vi "EnFlo_Data_Sync_Manual.vi"() -> ()   [LabVIEW 2013]
uses:
  Anemometry Sub Vis/Controls/EnFlo_Data_Folder_Setup.ctl
  ADAM Client/Sub VIs/Harvest_Global.vi
  Anemometry Sub Vis/Globals/Preference_global.vi
  Anemometry Sub Vis/Globals/Constants_global.vi
panel:
  in  "stop":bool
  out "Currrently Pulled":i32
  out "No Files to Push":i32
  out "No Files to Pull":i32
  out "Currrently Pushed":i32
  out "File being transfered":path
  out "Currently":string
  out "Files to Pull From Server":path[](array[path])
  out "Files to Push to Server":path[](array[path])
  in  "Browse Remote Disk":bool
  out "error out":errorcluster
  out "Folder contents changed?":bool
  in  "Folder to Sync (Must be within Local EnFlo Data)":path=path "C:/EnFlo_Data_Temp/EnFlo_Software_SVN"
  in  "Get all Server Files":bool
  in  "Check Updates on Server?":bool
  in  "Archive Files?":bool
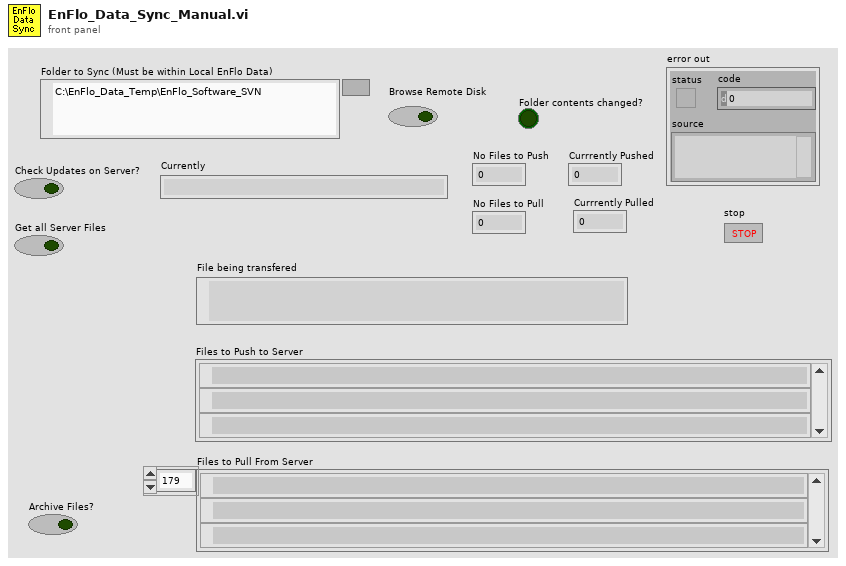
[diagram p1: front panel]
types:
  T1 = typedef "EnFlo_Data_Folder_Setup.ctl" = string
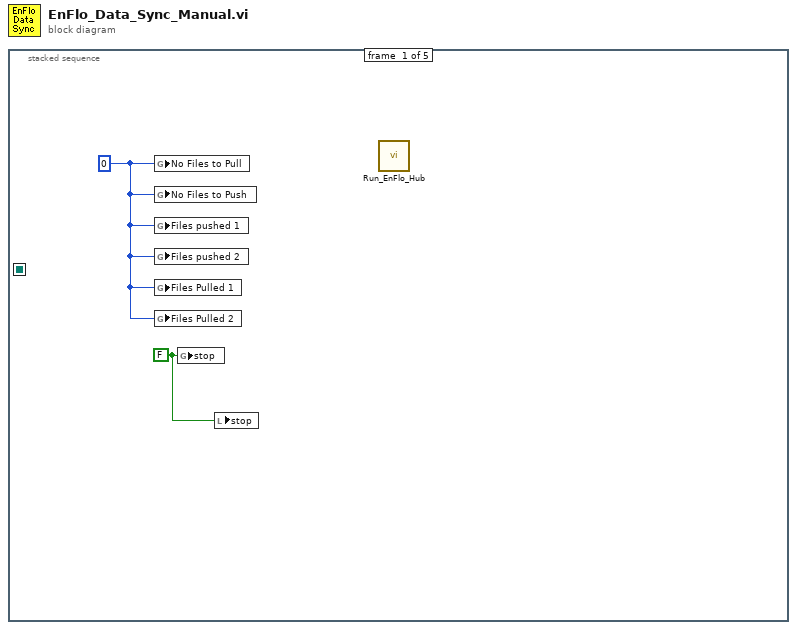
[diagram p0: block diagram]
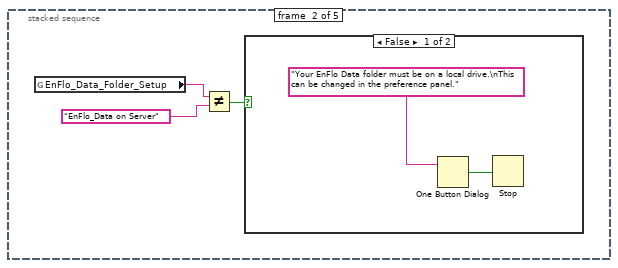
[diagram p2: hidden frame]
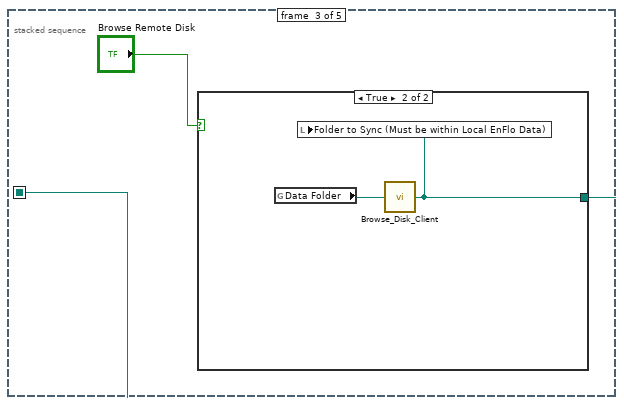
[diagram p4: hidden frame]
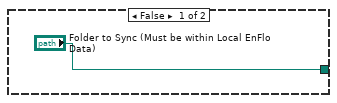
[diagram p5: hidden frame]
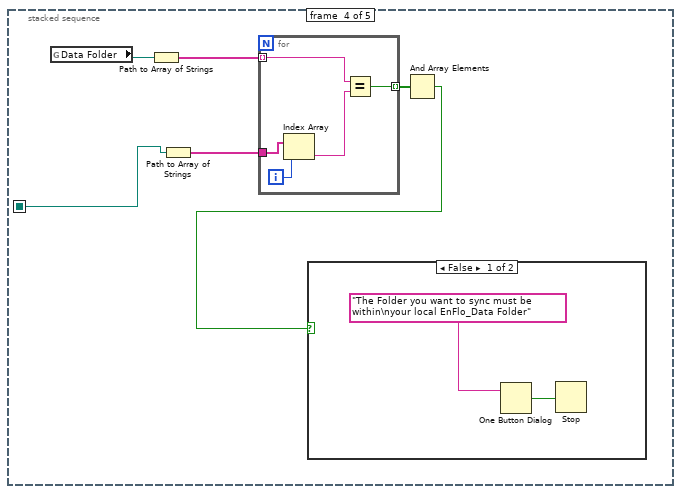
[diagram p6: hidden frame]
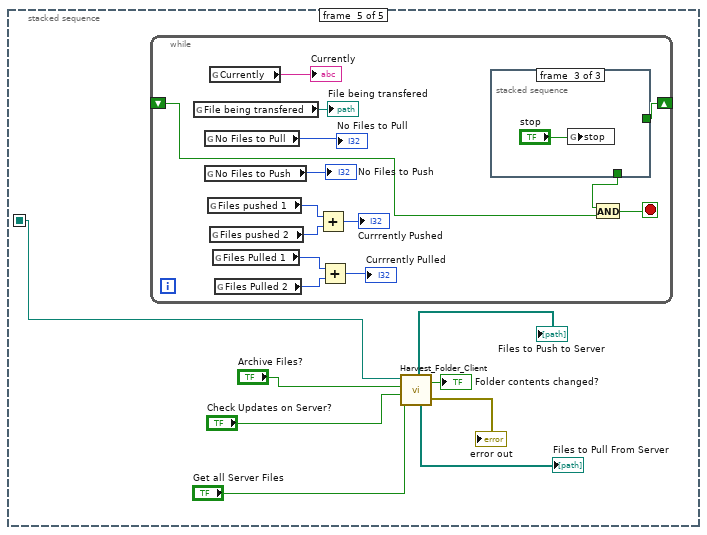
[diagram p8: hidden frame]
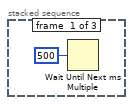
[diagram p9: hidden frame]
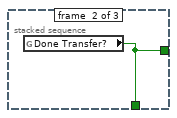
[diagram p10: hidden frame]
diagram:
  n1 = stacked-sequence {
    seq-local: [_ _ w8 _ _] -> [_ _ _ w13 w28]
    frame #0 {
      w1 = FALSE ("stop")
      w2 = 0 ("No Files to Pull")
      n2 = global write "Harvest_Global.vi" "No Files to Pull"(w2) -> ()
      n3 = global write "Harvest_Global.vi" "No Files to Push"(w2) -> ()
      n4 = global write "Harvest_Global.vi" "Files pushed 1"(w2) -> ()
      n5 = global write "Harvest_Global.vi" "Files pushed 2"(w2) -> ()
      n6 = global write "Harvest_Global.vi" "Files Pulled 1"(w2) -> ()
      n7 = global write "Harvest_Global.vi" "Files Pulled 2"(w2) -> ()
      n8 = global write "Harvest_Global.vi" "stop"(w1) -> ()
      n9 = local write "stop"(w1) -> ()
      n10 = call "Run_EnFlo_Hub.vi"() -> ()  [unwired: 8 in]
    }
    frame #1 {
      n11 = global read "Preference_global.vi" "EnFlo_Data_Folder_Setup"() -> (w4:T1)
      n12 = Not Equal?(x=w4, y=T1 "EnFlo_Data on Server" ("EnFlo_Data_Folder_Setup")) -> (x != y?=w5:bool)
      n13 = case shown="False" w5 {
        frame False {
          n14 = One Button Dialog(message="Your EnFlo Data folder must be on a local drive.\nThis can be changed in the preference panel.") -> (true=w6:bool)  [unwired: 1 in]
          n15 = Stop(stop? (T)=w6) -> ()
        }
        frame True {
        }
      }
    }
    frame #2 {
      n16 = case shown="True" "Browse Remote Disk" {
        tunnel: ["Folder to Sync (Must be within Local EnFlo Data)" w11] -> w8
        frame False {
        }
        frame True {
          n17 = global read "Constants_global.vi" "Data Folder"() -> (w12:path)
          n18 = call "Browse_Disk_Client.vi"("Start Path"=w12) -> ("Folder to Pull from Server"=w11:path)
          n19 = local write "Folder to Sync (Must be within Local EnFlo Data)"(w11) -> ()
        }
      }
    }
    frame #3 {
      n20 = global read "Constants_global.vi" "Data Folder"() -> (w18:path)
      n21 = Path to Array of Strings(0:w18) -> (2:w16:string[])  [unwired: 1 out]
      n22 = Path to Array of Strings(0:w13) -> (2:w17:string[])  [unwired: 1 out]
      n23 = for {
        tunnel: w17 -> [w23]
        tunnel: w16 -> [w21] mode=indexing
        tunnel: [w19] -> w15 mode=indexing
        i -> [w22]
        n24 = Index Array(array=w23, index=w22) -> (element=w20:string)
        n25 = Equal?(x=w21, y=w20) -> (x = y?=w19:bool)
      }
      n26 = And Array Elements(Boolean array=w15) -> (logical AND=w14:bool)
      n27 = case shown="False" w14 {
        frame False {
          n28 = One Button Dialog(message="The Folder you want to sync must be within\nyour local EnFlo_Data Folder") -> (true=w24:bool)  [unwired: 1 in]
          n29 = Stop(stop? (T)=w24) -> ()
        }
        frame True {
        }
      }
    }
    frame #4 {
      n30 = while {
        shift-right: [w37] -> _
        shift-left: _ -> [w34]
        stop <- w36 stop-if-true
        n31 = global read "Harvest_Global.vi" "File being transfered"() -> (→"File being transfered":path)
        n32 = global read "Harvest_Global.vi" "No Files to Pull"() -> (→"No Files to Pull":i32)
        n33 = global read "Harvest_Global.vi" "No Files to Push"() -> (→"No Files to Push":i32)
        n34 = global read "Harvest_Global.vi" "Files pushed 1"() -> (w42:i32)
        n35 = global read "Harvest_Global.vi" "Currently"() -> (→"Currently":string)
        n36 = global read "Harvest_Global.vi" "Files pushed 2"() -> (w43:i32)
        n37 = global read "Harvest_Global.vi" "Files Pulled 1"() -> (w40:i32)
        n38 = global read "Harvest_Global.vi" "Files Pulled 2"() -> (w39:i32)
        n39 = Add(x=w42, y=w43) -> (x+y=→"Currrently Pushed":i32)
        n40 = Add(x=w40, y=w39) -> (x+y=→"Currrently Pulled":i32)
        n41 = stacked-sequence {
          tunnel: [_ w49 _] -> w35
          tunnel: [_ w49 _] -> w37
          frame #0 {
            n42 = Wait Until Next ms Multiple(millisecond multiple=u32 500) -> ()  [unwired: 1 out]
          }
          frame #1 {
            n43 = global read "Harvest_Global.vi" "Done Transfer?"() -> (w49:bool)
          }
          frame #2 {
            n44 = global write "Harvest_Global.vi" "stop"("stop") -> ()
          }
        }
        n45 = And(x=w35, y=w34) -> (x .and. y?=w36:bool)
      }
      n46 = call "Harvest_Folder_Client.vi"("Get all Server Files"="Get all Server Files", "Check Updates on Server?"="Check Updates on Server?", "Archive Files?"="Archive Files?", "Folder to Harvest"=w28) -> ("error out"=→"error out":errorcluster, "Folder contents changed?"=→"Folder contents changed?":bool, "Files to Pull From Server"=→"Files to Pull From Server":path[], "Files to Push to Server"=→"Files to Push to Server":path[])
    }
  }
